vi "rect_scanning_cluster_fixed.vi"(9 "Slow Axis":i32, 10 "Fast Axis":i32, 11 "Scanning":T1={"Fast Axis Offset"=0.0, "Slow Axis Offset"=0.0, "Slow Axis Amp"=2.0, "Fast Axis Amp"=2.0, "Scan Pattern"=enum."Raster"} {"Fast Axis Amp" max=20 format="%#.2f"; "Slow Axis Amp" max=20 format="%#.2f"; "Slow Axis Offset" max=10 format="%#.2f"; "Fast Axis Offset" max=10 format="%#.2f"}) -> (3 "Scan Pattern 7":dbl[][](graph))   [LabVIEW 2015, in "Galvo.lvclass"]
uses:
  Galvo.lvclass
  Scanning Cluster.ctl
  <vilib>/Analysis/NI_AALBase.lvlib
panel:
  out "Scan Pattern":cluster{dbl[], dbl[]}(graph)
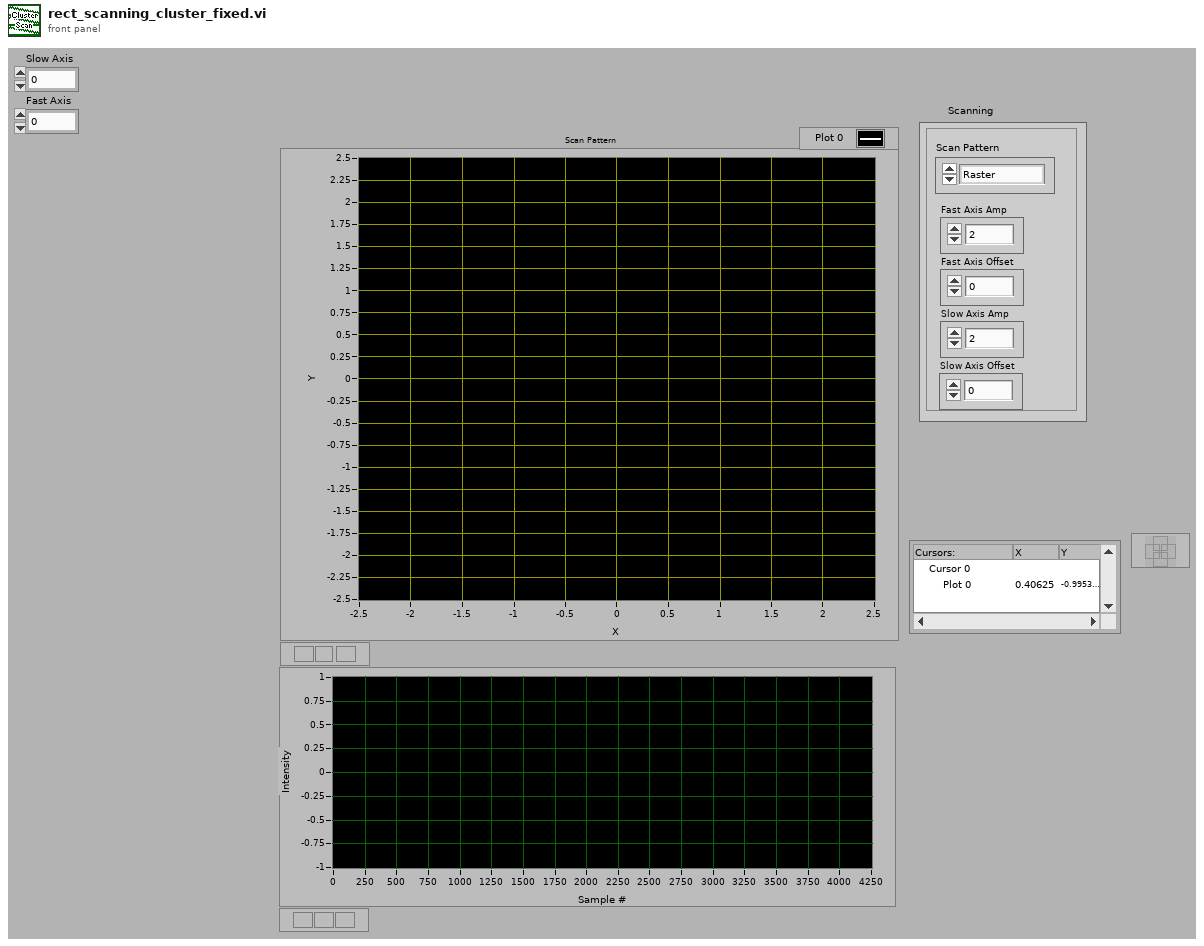
[diagram p1: front panel]
types:
  T1 = typedef "Galvo.lvclass/Scanning Cluster.ctl" = cluster{"Fast Axis Offset":sgl, "Slow Axis Offset":sgl, "Slow Axis Amp":sgl, "Fast Axis Amp":sgl, "Scan Pattern":enum16{"Raster", "Triangle Raster", "Sinusoid Raster"}}
  T2 = enum16{"Raster", "Triangle Raster", "Sinusoid Raster"}
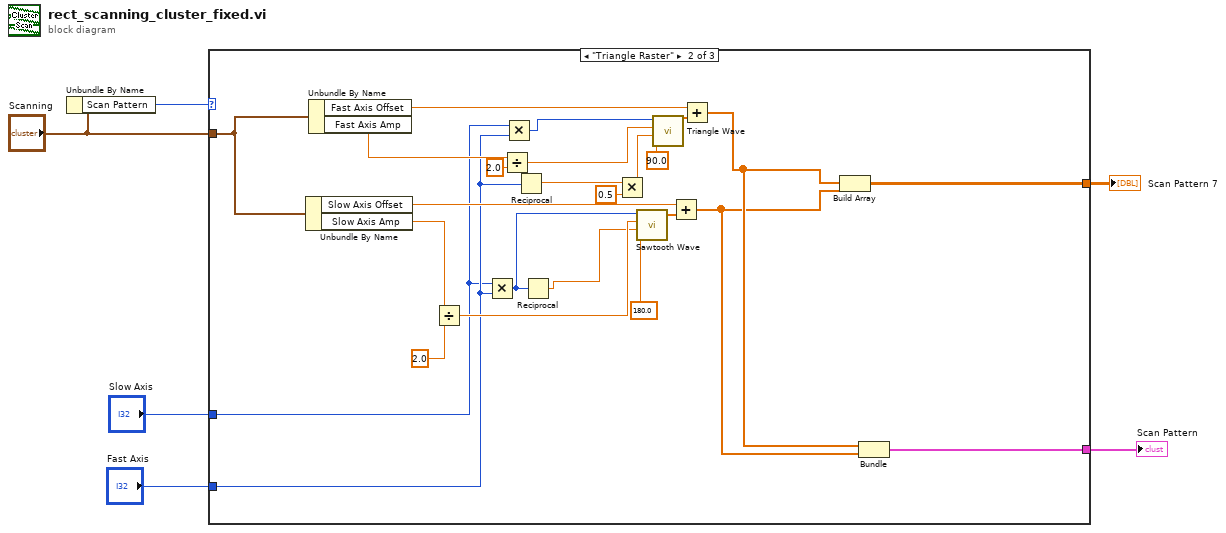
[diagram p0: block diagram]
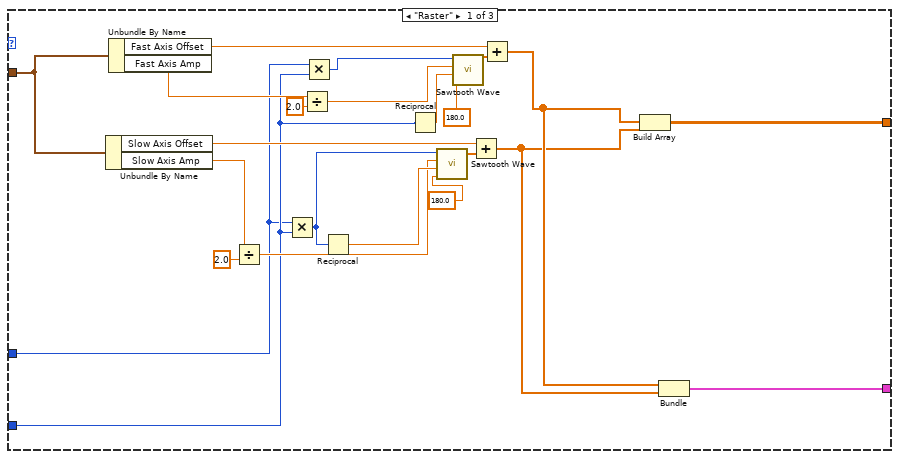
[diagram p2: hidden frame]
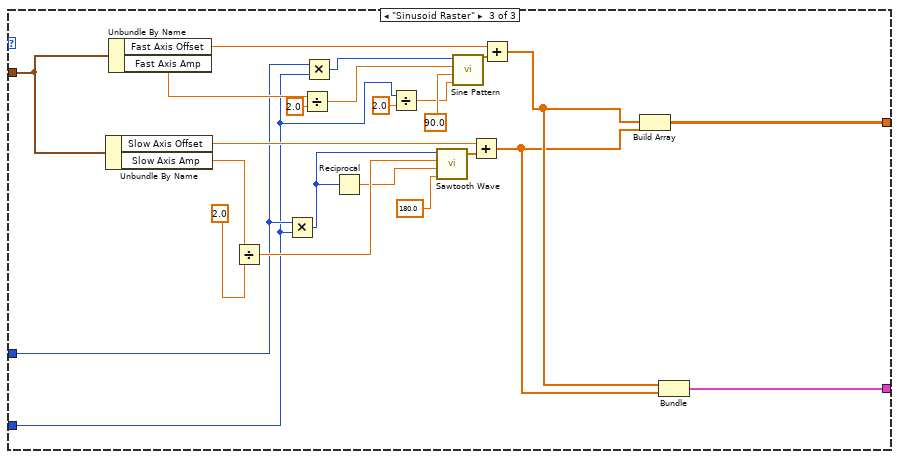
[diagram p3: hidden frame]
diagram:
  n1 = Unbundle By Name("Scanning") -> ("Scan Pattern"=w3:T2)
  n2 = case shown="\"Triangle Raster\"" w3 {
    tunnel: "Scanning" -> [w16 w43 w69]
    tunnel: [w13 w40 w66] -> w6
    tunnel: [w12 w39 w65] -> w5
    tunnel: "Slow Axis" -> [w8 w35 w62]
    tunnel: "Fast Axis" -> [w9 w36 w57]
    frame "Raster" {
      n3 = Unbundle By Name(w16) -> ("Slow Axis Offset"=w11:sgl, "Slow Axis Amp"=w20:sgl)
      n4 = Unbundle By Name(w16) -> ("Fast Axis Offset"=w21:sgl, "Fast Axis Amp"=w23:sgl)
      n5 = Divide(x=w20, y=2.0) -> (x/y=w15:dbl)
      n6 = Multiply(x=w8, y=w9) -> (x*y=w7:i32)
      n7 = Divide(x=w23, y=2.0 ("x")) -> (x/y=w10:dbl)
      n8 = Multiply(x=w8, y=w9) -> (x*y=w22:i32)
      n9 = Reciprocal(x=w7) -> (1/x=w26:dbl)
      n10 = Reciprocal(x=w9) -> (1/x=w25:dbl)
      n11 = call <vilib>:"Sawtooth Wave.vi"("samples"=w7, "amplitude"=w15, "frequency"=w26, "phase in"=180.0 ("S_phase")) -> ("sawtooth wave"=w28:dbl[])  [unwired: 1 in, 2 out]
      n12 = call <vilib>:"Sawtooth Wave.vi"("samples"=w22, "amplitude"=w10, "frequency"=w25, "phase in"=180.0) -> ("sawtooth wave"=w29:dbl[])  [unwired: 1 in, 2 out]
      n13 = Add(x=w11, y=w28) -> (x+y=w18:dbl[])
      n14 = Add(x=w21, y=w29) -> (x+y=w19:dbl[])
      n15 = Build Array(w19, w18) -> (w12:dbl[][])
      n16 = Bundle(w19, w18) -> (w13:cluster{dbl[], dbl[]})  [unwired: 1 out]
    }
    frame "Triangle Raster" {
      n17 = Unbundle By Name(w43) -> ("Slow Axis Offset"=w38:sgl, "Slow Axis Amp"=w47:sgl)
      n18 = Unbundle By Name(w43) -> ("Fast Axis Offset"=w48:sgl, "Fast Axis Amp"=w50:sgl)
      n19 = Divide(x=w47, y=2.0) -> (x/y=w42:dbl)
      n20 = Multiply(x=w35, y=w36) -> (x*y=w34:i32)
      n21 = Divide(x=w50, y=2.0 ("x")) -> (x/y=w37:dbl)
      n22 = Multiply(x=w35, y=w36) -> (x*y=w49:i32)
      n23 = Reciprocal(x=w36) -> (1/x=w33:dbl)
      n24 = Reciprocal(x=w34) -> (1/x=w30:dbl)
      n25 = Multiply(x=w33, y=0.5 ("x")) -> (x*y=w32:dbl)
      n26 = call <vilib>:"Sawtooth Wave.vi"("samples"=w34, "amplitude"=w42, "frequency"=w30, "phase in"=180.0 ("S_phase")) -> ("sawtooth wave"=w53:dbl[])  [unwired: 1 in, 2 out]
      n27 = call <vilib>:"Triangle Wave.vi"("samples"=w49, "amplitude"=w37, "frequency"=w32, "phase in"=90.0) -> ("triangle wave"=w54:dbl[])  [unwired: 1 in, 2 out]
      n28 = Add(x=w38, y=w53) -> (x+y=w45:dbl[])
      n29 = Add(x=w48, y=w54) -> (x+y=w46:dbl[])
      n30 = Build Array(w46, w45) -> (w39:dbl[][])
      n31 = Bundle(w46, w45) -> (w40:cluster{dbl[], dbl[]})  [unwired: 1 out]
    }
    frame "Sinusoid Raster" {
      n32 = Unbundle By Name(w69) -> ("Slow Axis Offset"=w64:sgl, "Slow Axis Amp"=w73:sgl)
      n33 = Unbundle By Name(w69) -> ("Fast Axis Offset"=w74:sgl, "Fast Axis Amp"=w76:sgl)
      n34 = Divide(x=w73, y=2.0) -> (x/y=w68:dbl)
      n35 = Multiply(x=w62, y=w57) -> (x*y=w60:i32)
      n36 = Divide(x=w76, y=2.0 ("x")) -> (x/y=w63:dbl)
      n37 = Multiply(x=w62, y=w57) -> (x*y=w75:i32)
      n38 = Reciprocal(x=w60) -> (1/x=w59:dbl)
      n39 = Divide(x=w57, y=2.0 ("x")) -> (x/y=w56:dbl)
      n40 = call <vilib>:"Sawtooth Wave.vi"("samples"=w60, "amplitude"=w68, "frequency"=w59, "phase in"=180.0 ("S_phase")) -> ("sawtooth wave"=w77:dbl[])  [unwired: 1 in, 2 out]
      n41 = call <vilib>:"Sine Pattern.vi"("cycles"=w56, "phase(degrees)"=90.0 ("phase in"), "amplitude"=w63, "samples"=w75) -> ("Sinusoidal Pattern"=w78:dbl[])  [unwired: 1 out]
      n42 = Add(x=w64, y=w77) -> (x+y=w71:dbl[])
      n43 = Add(x=w74, y=w78) -> (x+y=w72:dbl[])
      n44 = Build Array(w72, w71) -> (w65:dbl[][])
      n45 = Bundle(w72, w71) -> (w66:cluster{dbl[], dbl[]})  [unwired: 1 out]
    }
  }
  "Scan Pattern 7" <- w5
  "Scan Pattern" <- w6
